vi "SP.vi"(1 "Ctl Refnum 2":refnum<vi>, 2 "Ctl Refnum":refnum<vi>, 5 "表格（SP）路径：":path=path "C:/Users/shipeng/Desktop/Z-f Dielectric measurement LOG RT", 6 "时间间隔(s)":dbl=2.0, 7 "开始频率":dbl[](array[numeric])=[20.0, 5000000.0, 100.0], 8 "error in (no error)":errorcluster caption="错误输入（无错误）", 9 "客户仪器地址":refnum<visa-resource-name>="USB0::0x0471::0x2826::QF71600867::INSTR", 10 "Scanning Mode":u16(ring)=1 items=["Linear", "Log"], 11 "文本（SP）路径：":path=path "C:/Users/shipeng/Desktop/Z-f Dielectric measurement LOG RT") -> (0 "错误输出":cluster{"状态":bool, "代码":i32, "源":string})   [LabVIEW 2017]
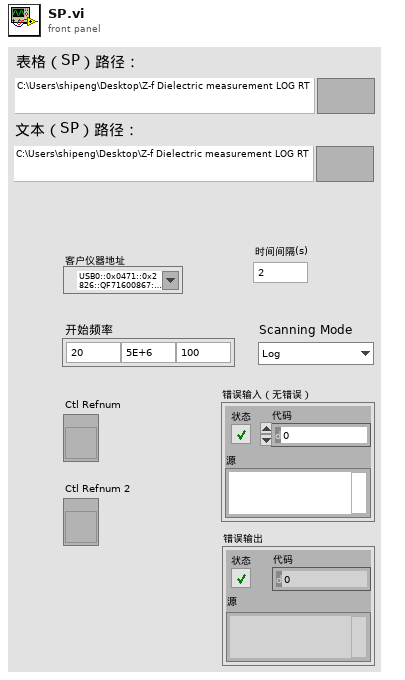
[diagram p1: front panel]
types:
  T1 = enum16{"open", "replace", "create", "open or create", "replace or create", "replace or create with confirmation"}
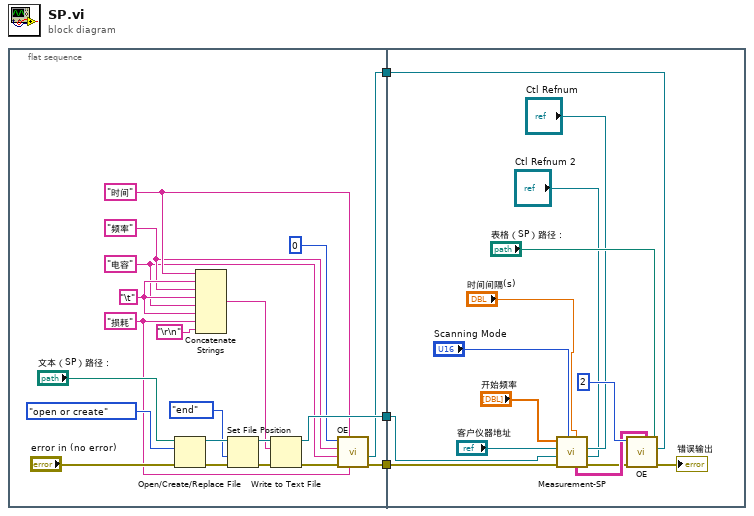
[diagram p0: block diagram]
diagram:
  n1 = flat-sequence {
    tunnel: [w14] -> w3
    tunnel: [w5] -> w2
    tunnel: [w4] -> w1
    tunnel: w3 -> [w36]
    tunnel: w2 -> [w35]
    tunnel: w1 -> [w29]
    frame #0 {
      w7 = "损耗" ("字符串")
      w8 = "电容" ("字符串")
      w9 = "频率" ("字符串")
      w16 = "\t"
      w10 = "时间" ("字符串")
      n2 = Open/Create/Replace File(file path (use dialog)="文本（SP）路径：", error in="error in (no error)", operation (0:open)=T1."open or create" ("操作(0:open)")) -> (refnum out=w21:refnum<file>, error out=w18:errorcluster)  [unwired: 4 out]
      n3 = Concatenate Strings(w10, w16, w9, w16, w8, w16, w7, "\r\n") -> (w17:string)
      n4 = Set File Position(refnum=w21, from (0:start)=enum16{"start", "end", "current"}."end" ("自（0:起始）"), error in=w18) -> (refnum out=w22:refnum<file>, error out=w23:errorcluster)  [unwired: 1 out]
      n5 = Write to Text File(file (use dialog)=w22, text=w17, error in=w23) -> (refnum out=w14:refnum<file>, error out=w6:errorcluster)  [unwired: 2 out]
      n6 = call "OE.vi"("String 4"=w7, "String"=w10, "error in (no error)"=w6, "String 3"=w8, "String 2"=w9, "Numeric"=0) -> ("error out"=w5:errorcluster, "report out"=w4:refnum<class "NI_report.lvclass">)  [unwired: 3 in, 1 out]
    }
    frame #1 {
      n7 = call "Measurement-SP.vi"("Ctl Refnum 2"="Ctl Refnum 2", "Ctl Refnum"="Ctl Refnum", "时间间隔"="时间间隔(s)", "Scanning Mode"="Scanning Mode", "error in (no error)"=w35, "Byte Stream File Refnum"=w36, "客户仪器地址"="客户仪器地址", "开始频率"="开始频率") -> ("error out"=w27:errorcluster, "Array"=w30:string[][])  [unwired: 2 in]
      n8 = call "OE.vi"("report in"=w29, "表格数据路径："="表格（SP）路径：", "Array"=w30, "error in (no error)"=w27, "Numeric"=2) -> ("error out"=→"错误输出":errorcluster)  [unwired: 4 in, 2 out]
    }
  }
